vi "Experiment header-Save_Load CAL section.vi"(8 "error in (no error)":errorcluster, 10 "Function":enum16{"Write", "Read"}(ring), 11 "Experiment folder path":path) -> (0 "error out":errorcluster, 3 "Cal file names from test header file":string[](array[string]))   [LabVIEW 2017]
uses:
  Configuration code/Calibration/Globals/gl_Calibration globals.vi
  <vilib>/Utility/config.llb/Read Key (String).vi
  <vilib>/Utility/config.llb/Write Key (String).vi
  <vilib>/Utility/config.llb/NI_LVConfig.lvlib
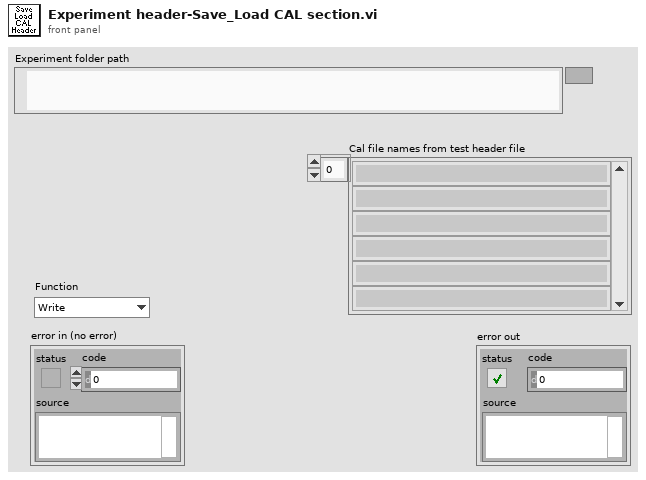
[diagram p1: front panel]
types:
  T1 = typedef "Fixed strings.ctl" = cluster{"ROI file name":string, "Normalised ROI file name":string, "Zplane Pockels values file name":string, "Functional data folder name":string, "Experiment Header file name":string, "Z-stack images folder name":string, "Groups setup rel. path":string, "Groups text file rel. path":string, "TDMS files folder name (F.img)":string, "TDMS files folder name (V.acq)":string, "TDMS files folder name (Pl.acq)":string, "Cycle rel times sequence file":string, "Dynamically called VIs folder name":string, "Time Series folder base name":string}
  T2 = typedef "NI_LVConfig.lvlib/Config Data RefNum.ctl" = refnum<k1>
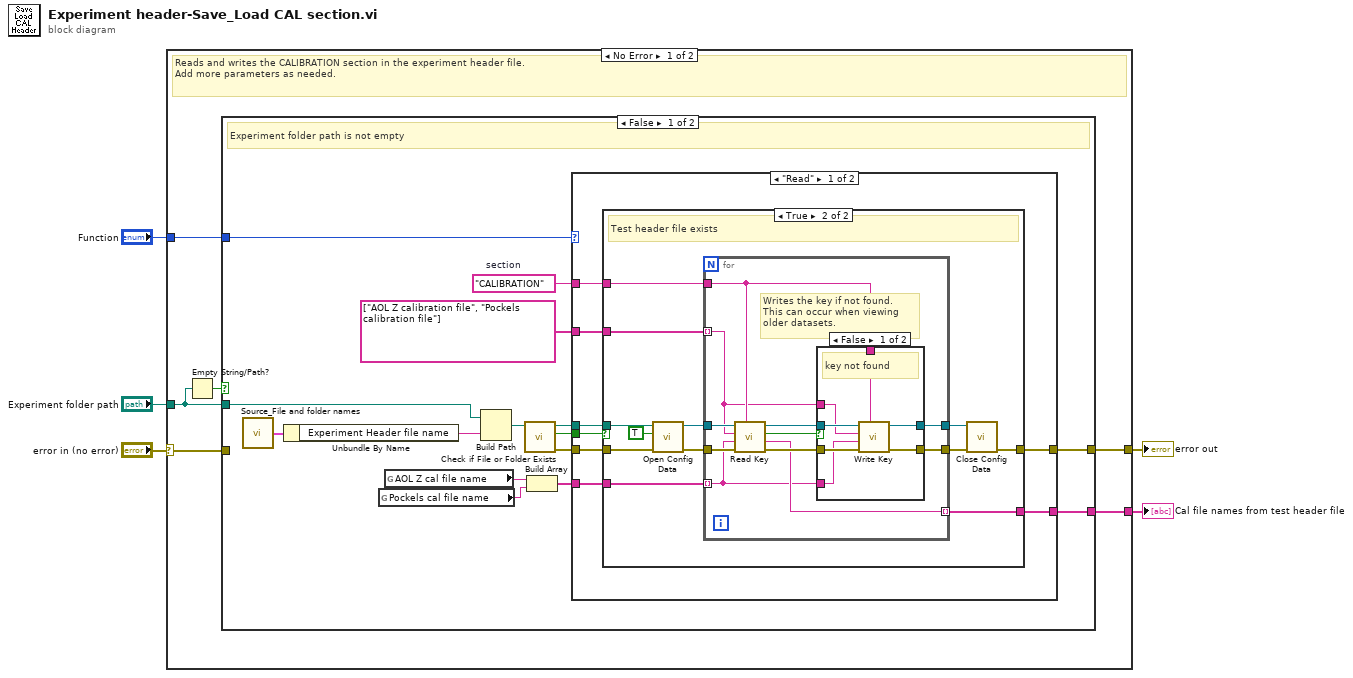
[diagram p0: block diagram]
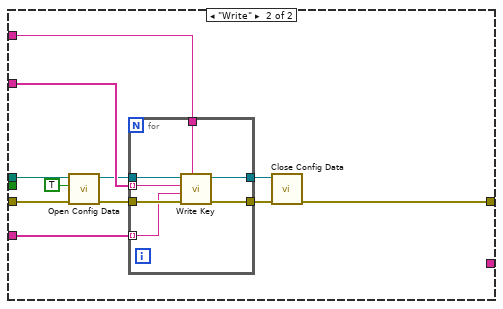
[diagram p4: hidden frame]
diagram:
  n1 = case shown="No Error" "error in (no error)" {
    selector: "error in (no error)" -> [w7 w87]
    tunnel: [w11 w87] -> w5
    tunnel: "Function" -> [w10 _]
    tunnel: "Experiment folder path" -> [w8 _]
    tunnel: [w6 _] -> w1
    frame No Error {
      # "Reads and writes the CALIBRATION section in the experiment header file.\nAdd more parameters as needed."
      n2 = Empty String/Path?(string/path=w8) -> (empty?=w9:bool)
      n3 = case shown="False" w9 {
        tunnel: [w16 w86] -> w11
        tunnel: w10 -> [w20 _]
        tunnel: w8 -> [w21 _]
        tunnel: w7 -> [_ w86]
        tunnel: [w14 _] -> w6
        frame False {
          w22 = "CALIBRATION"  # section
          # "Experiment folder path is not empty"
          n4 = call "Source_File and folder names.vi"() -> ("Fixed strings"=w24:T1)  [unwired: 1 in]
          n5 = Unbundle By Name(w24) -> ("Experiment Header file name"=w25:string)
          n6 = global read "gl_Calibration globals.vi" "Pockels cal file name"() -> (w12:string)
          n7 = global read "gl_Calibration globals.vi" "AOL Z cal file name"() -> (w13:string)
          n8 = Build Path(base path=w21, name or relative path=w25) -> (appended path=w23:path)
          n9 = call <vilib>:"Check if File or Folder Exists.vi"("path"=w23) -> ("error out"=w17:errorcluster, "file or folder exists?"=w19:bool, "dup path"=w18:path)  [unwired: 8 in]
          n10 = Build Array(w13, w12) -> (w15:string[])
          n11 = case shown="\"Read\"" w20 {
            tunnel: [w33 w70] -> w16
            tunnel: w17 -> [w34 w74]
            tunnel: w22 -> [w32 w78]
            tunnel: string[] ["AOL Z calibration file", "Pockels calibration file"] -> [w31 w77]
            tunnel: w19 -> [w29 _]
            tunnel: w18 -> [w30 w75]
            tunnel: w15 -> [w28 w68]
            tunnel: [w27 _] -> w14
            frame "Read" {
              n12 = case shown="True" w29 {
                tunnel: w34 -> [w35 w42]
                tunnel: [w35 w38] -> w33
                tunnel: w32 -> [_ w47]
                tunnel: w31 -> [_ w46]
                tunnel: w30 -> [_ w45]
                tunnel: w28 -> [_ w37]
                tunnel: [_ w36] -> w27
                frame False {
                  # "Test header file doesnot exist"
                }
                frame True {
                  # "Test header file exists"
                  n13 = call <vilib>:"Open Config Data.vi"("error in (no error)"=w42, "create file if necessary (T)"=TRUE, "configuration file path"=w45) -> ("error out"=w41:errorcluster, "refnum"=w43:T2)  [unwired: 6 in, 1 out]
                  n14 = for {
                    tunnel: w43 -> [w58]
                    tunnel: w41 -> [w57]
                    tunnel: [w54] -> w40
                    tunnel: [w53] -> w39
                    tunnel: w47 -> [w52]
                    tunnel: [w50] -> w36 mode=indexing
                    tunnel: w37 -> [w48] mode=indexing
                    tunnel: w46 -> [w49] mode=indexing
                    # "Writes the key if not found.\nThis can occur when viewing older datasets."
                    n15 = call-poly <vilib>:"Read Key.vi"("section"=w52, "error in (no error)"=w57, "default value"=w48, "key"=w49, "refnum"=w58) -> ("error out"=w55:errorcluster, "value"=w50:string, "found?"=w51:bool, "refnum out"=w56:T2)  [unwired: 3 in]
                    n16 = case shown="False" w51 {
                      tunnel: w56 -> [w65 w67]
                      tunnel: w55 -> [w64 w66]
                      tunnel: [w63 w67] -> w54
                      tunnel: [w62 w66] -> w53
                      tunnel: w52 -> [w61 _]
                      tunnel: w49 -> [w60 _]
                      tunnel: w48 -> [w59 _]
                      frame False {
                        # "key not found"
                        n17 = call-poly <vilib>:"Write Key.vi"("section"=w61, "error in (no error)"=w64, "value"=w59, "key"=w60, "refnum"=w65) -> ("error out"=w62:errorcluster, "refnum out"=w63:T2)  [unwired: 4 in, 1 out]
                      }
                      frame True {
                        # "found"
                      }
                    }
                  }
                  n18 = call <vilib>:"Close Config Data.vi"("error in (no error)"=w39, "refnum"=w40) -> ("error out"=w38:errorcluster)  [unwired: 8 in, 1 out]
                }
              }
            }
            frame "Write" {
              n19 = call <vilib>:"Open Config Data.vi"("error in (no error)"=w74, "create file if necessary (T)"=TRUE, "configuration file path"=w75) -> ("error out"=w73:errorcluster, "refnum"=w76:T2)  [unwired: 6 in, 1 out]
              n20 = for {
                tunnel: w76 -> [w85]
                tunnel: w73 -> [w84]
                tunnel: w77 -> [w83] mode=indexing
                tunnel: w78 -> [w82]
                tunnel: [w81] -> w69
                tunnel: [w80] -> w71
                tunnel: w68 -> [w79] mode=indexing
                n21 = call-poly <vilib>:"Write Key.vi"("section"=w82, "error in (no error)"=w84, "value"=w79, "key"=w83, "refnum"=w85) -> ("error out"=w81:errorcluster, "refnum out"=w80:T2)  [unwired: 4 in, 1 out]
              }
              n22 = call <vilib>:"Close Config Data.vi"("error in (no error)"=w69, "refnum"=w71) -> ("error out"=w70:errorcluster)  [unwired: 8 in, 1 out]
            }
          }
        }
        frame True {
          # "Empty experiment folder path path"
        }
      }
    }
    frame Error {
    }
  }
  "error out" <- w5
  "Cal file names from test header file" <- w1
